vi "Send Add Value without TS.vi"(0 "Message Enqueuer":refnum<class "Message Enqueuer.lvclass">, 1 "Value":dbl, 5 "error in (no error)":errorcluster, 6 "Actor Name":string, 7 "Callback Queue":refnum<queue>, 8 "Message Priority (Normal)":T1=enum."Normal", 9 "timeout in ms (-1)":i32) -> (13 "TimeOut":bool, 14 "Message Enqueuer out":refnum<class "Message Enqueuer.lvclass">, 19 "error out":errorcluster)   [LabVIEW 2018, in "BNT_XtGraph.lvlib" / "Add Value without TS Msg.lvclass"]
doc: "Sends the <B>BNT_XtGraph.lvlib:Add Value without TS Msg.lvclass</B> message.\n\n<B>BNT_XtGraph.lvlib:BNT_XtGraph.lvclass:Add Value without TS.vi</B> Description:\n\nAdd actual value with time <b>now</b> to history."
uses:
  Add Value without TS Msg.lvclass
  <vilib>/ActorFramework/Message Enqueuer/Message Enqueuer.lvclass
  <vilib>/ActorFramework/Message Enqueuer/Message Priority.ctl
  C:/Users/Holger/Documents/LVP/HEITRONICS/TempCtrl/Packages/CSPP_Core/Messages/CSPP_AsyncCallbackMsg/CSPP_AsyncCallback Msg.lvclass
  C:/Program Files (x86)/National Instruments/LabVIEW 2018/vi.lib/ActorFramework/Message/Message.lvclass
  Add Value without TS Msg.lvclass/Add Value without TS Msg.ctl
  CSPP_Core/Messages/CSPP_AsyncCallbackMsg/CSPP_AsyncCallback Msg.lvclass/CSPP_AsyncCallback Msg.ctl
  <vilib>/ActorFramework/Message Enqueuer/Message Enqueuer.lvclass/Message Enqueuer.ctl
  <vilib>/ActorFramework/Message Priority Queue/Priority Enqueue.vi
  CSPP_Core/Messages/CSPP_AsyncCallbackMsg/CSPP_AsyncCallback Msg.lvclass
  CSPP_Core/Libraries/Utilities/CSPP_Utilities.lvlib
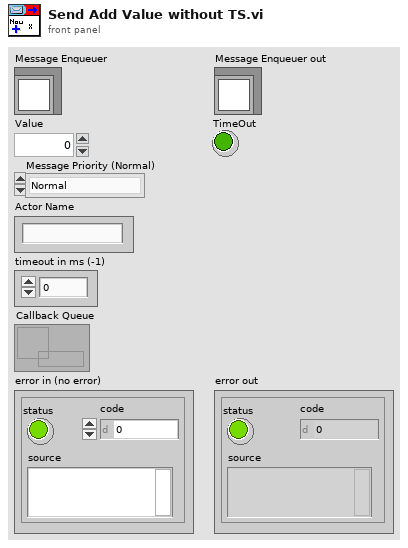
[diagram p1: front panel]
types:
  T1 = typedef "Actor Framework.lvlib/Message Enqueuer.lvclass/Message Priority.ctl" = enum16{"Low", "Normal", "High"}
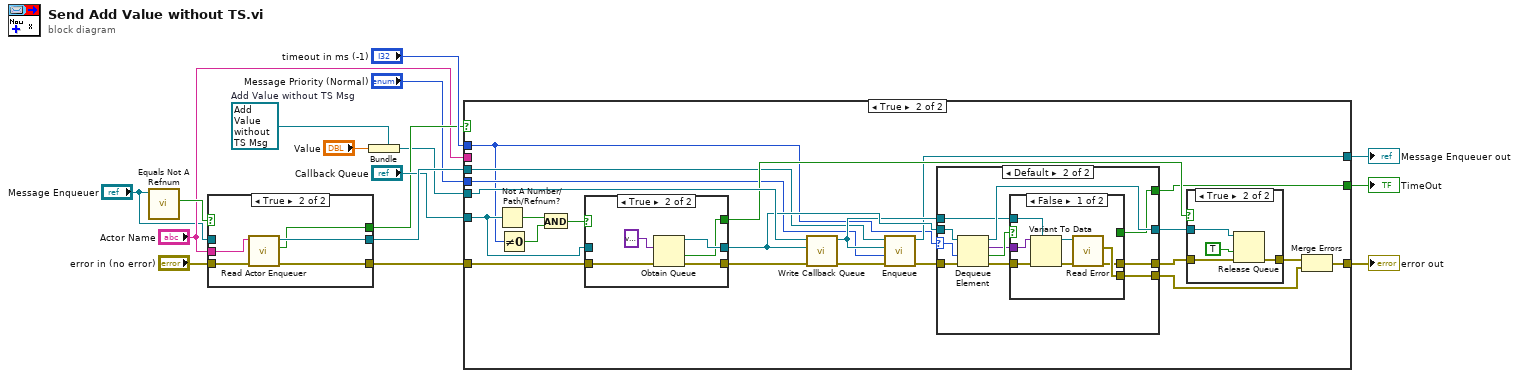
[diagram p0: block diagram]
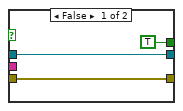
[diagram p2: hidden frame]
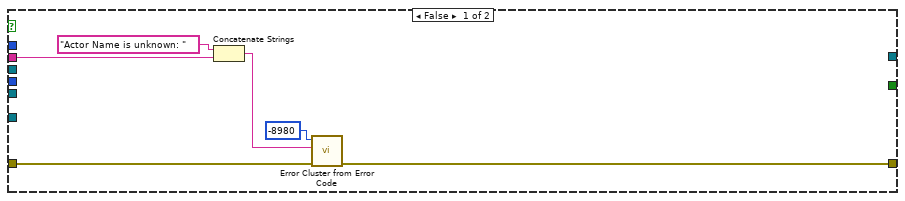
[diagram p3: hidden frame]
diagram:
  w3 = refnum<class "Add Value without TS Msg.lvclass"> refnum  # Add Value without TS Msg
  n1 = call <vilib>:"Equals Not A Refnum.vi"("Message Enqueuer"="Message Enqueuer") -> ("Not a refnum?"=w16:bool)  [unwired: 10 in]
  n2 = case shown="True" w16 {
    tunnel: "error in (no error)" -> [w18 w24]
    tunnel: [w18 w23] -> w15
    tunnel: "Actor Name" -> [_ w20]
    tunnel: [w19 w22] -> w14
    tunnel: "Message Enqueuer" -> [w19 _]
    tunnel: [TRUE ("Success") w21] -> w10
    frame False {
    }
    frame True {
      n3 = call "Read Actor Enqueuer.vi"("Error In"=w24, "Actor Name"=w20) -> ("Error Out"=w23:errorcluster, "Success"=w21:bool, "Enqueuer"=w22:refnum<class "Message Enqueuer.lvclass">)  [unwired: 6 in, 1 out]
    }
  }
  n4 = Bundle ("Main-Bundle")(cluster=w3, "Value") -> (w4:refnum<class "Add Value without TS Msg.lvclass">)
  n5 = case shown="True" w10 {
    tunnel: w4 -> [_ w52]
    tunnel: w15 -> [w30 w41]
    tunnel: w14 -> [_ w40]
    tunnel: "Message Priority (Normal)" -> [_ w39]
    tunnel: "Callback Queue" -> [_ w32]
    tunnel: [_ w38] -> w6
    tunnel: [w29 w37] -> w7
    tunnel: [_ w36] -> w12
    tunnel: "timeout in ms (-1)" -> [_ w31]
    tunnel: "Actor Name" -> [w25 _]
    frame False {
      n6 = Concatenate Strings("Actor Name is unknown: " ("Error Message (\"\")"), w25) -> (w26:string)
      n7 = call "Error Cluster from Error Code.vi"("Error In"=w30, "Error Message (\"\")"=w26, "Error Code (0)"=-8980) -> ("Error Out"=w29:errorcluster)  [unwired: 8 in]
    }
    frame True {
      n8 = Not A Number/Path/Refnum?(number/path/refnum=w32) -> (NaN/Path/Refnum?=w35:bool)
      n9 = Not Equal To 0?(x=w31) -> (x != 0?=w34:bool)
      n10 = And(x=w35, y=w34) -> (x .and. y?=w33:bool)
      n11 = case shown="True" w33 {
        tunnel: w32 -> [w76 _]
        tunnel: [w76 w81] -> w49
        tunnel: [w75 w79] -> w50
        tunnel: w41 -> [w75 w78]
        tunnel: [_ w77] -> w47
        frame False {
        }
        frame True {
          n12 = Obtain Queue(element data type=variant, error in (no error)=w78) -> (queue out=w81:refnum<queue>, created new?=w77:bool, error out=w79:errorcluster)  [unwired: 3 in]
        }
      }
      n13 = call "Write Callback Queue.vi"("error in (no error)"=w50, "Callback Queue"=w49, "CSPP_AsyncCallback Msg in"=w52) -> ("error out"=w51:errorcluster, "CSPP_AsyncCallback Msg out"=w43:refnum<class "Add Value without TS Msg.lvclass">)  [unwired: 7 in]
      n14 = call <vilib>:"Enqueue.vi"("error in (no error)"=w51, "Message Priority (Normal)"=w39, "Message"=w43, "Message Enqueuer in"=w40) -> ("error out"=w48:errorcluster, "Message Enqueuer out"=w38:refnum<class "Message Enqueuer.lvclass">)  [unwired: 6 in]
      n15 = case shown="Default" w31 {
        selector: w31 -> [_ w62]
        tunnel: w49 -> [w54 w63]
        tunnel: [w54 w65] -> w46
        tunnel: [w53 w55] -> w45
        tunnel: w48 -> [w53 w64]
        tunnel: w43 -> [_ w59]
        tunnel: [_ w57] -> w36
        tunnel: [_ w56] -> w42
        frame 0 {
        }
        frame Default {
          n16 = Dequeue Element(queue=w63, timeout in ms (-1)=w62, error in (no error)=w64) -> (queue out=w65:refnum<queue>, element=w60:variant, timed out?=w61:bool, error out=w58:errorcluster)
          n17 = case "Dequeue Case" shown="False" w61 {
            selector: w61 -> [_ w74]
            tunnel: w60 -> [w72 _]
            tunnel: w59 -> [w71 _]
            tunnel: w58 -> [w70 w73]
            tunnel: [_ w74] -> w57
            tunnel: [w67 _] -> w56
            tunnel: [w66 w73] -> w55
            frame False {
              n18 = Variant To Data(error in=w70, type=w71, Variant=w72) -> (data=w69:refnum<class "Add Value without TS Msg.lvclass">, error out=w68:errorcluster)
              n19 = call "Read Error.vi"("error in (no error)"=w68, "CSPP_AsyncCallback Msg in"=w69) -> ("error out"=w66:errorcluster, "Error"=w67:errorcluster)  [unwired: 7 in, 1 out]
            }
            frame True {
            }
          }
        }
      }
      n20 = case shown="True" w47 {
        tunnel: w46 -> [_ w86]
        tunnel: w45 -> [w82 w85]
        tunnel: [w82 w83] -> w44
        frame False {
        }
        frame True {
          n21 = Release Queue(queue=w86, force destroy? (F)=TRUE, error in (no error)=w85) -> (error out=w83:errorcluster)  [unwired: 2 out]
        }
      }
      n22 = Merge Errors(w44, w42) -> (w37:errorcluster)
    }
  }
  "error out" <- w7
  "Message Enqueuer out" <- w6
  "TimeOut" <- w12
